vi "Read.vi"(8 "error in":errorcluster, 11 "Channel":u16) -> (0 "error out":errorcluster, 2 "MessageBuffer out":T1, 3 "Channel out":u16, 5 "function return":u32)   [LabVIEW 2025, in "PCAN API.lvlib"]
doc: "This VI is used for reading a CAN message with decoding errors from function return."
uses:
  PCAN API.lvlib
  <vilib>/Utility/file.llb/Write Delimited Spreadsheet (string).vi
  PCAN2023/PCAN2023.lvlib
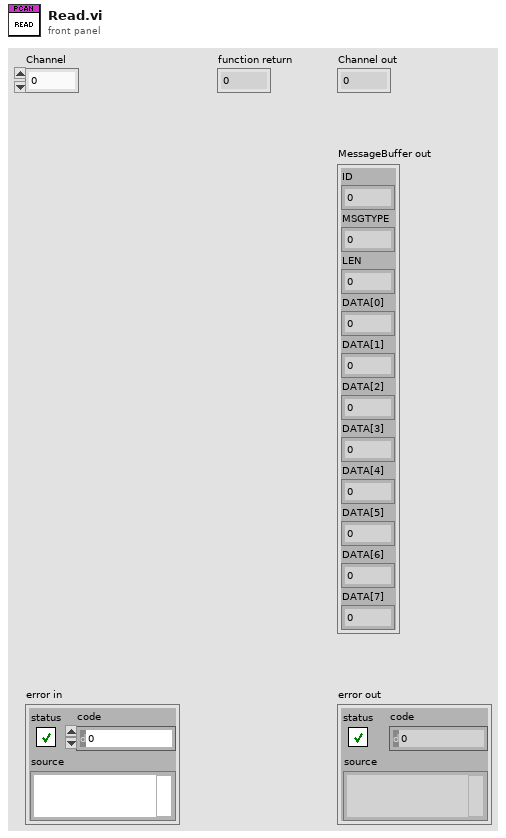
[diagram p1: front panel]
types:
  T1 = cluster{"ID":u32, "MSGTYPE":u8, "LEN":u8, "DATA[0]":u8, "DATA[1]":u8, "DATA[2]":u8, "DATA[3]":u8, "DATA[4]":u8, "DATA[5]":u8, "DATA[6]":u8, "DATA[7]":u8}
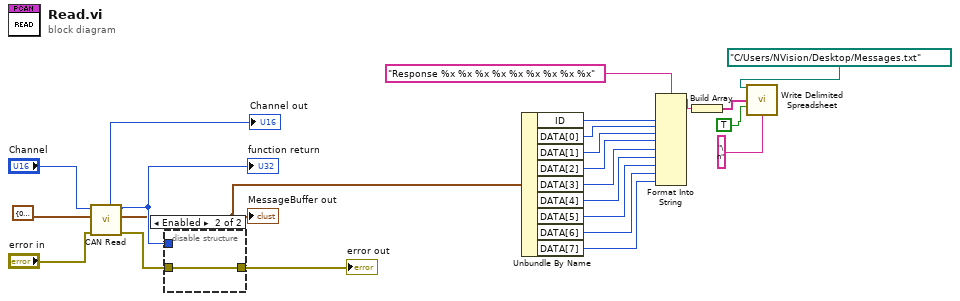
[diagram p0: block diagram]
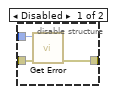
[diagram p2: hidden frame]
diagram:
  n1 = call "CAN Read.vi"("error in"="error in", "MessageBuffer"=T1 {"ID"=0, "MSGTYPE"=0, "LEN"=0, "DATA[0]"=0, "DATA[1]"=0, "DATA[2]"=0, "DATA[3]"=0, "DATA[4]"=0, "DATA[5]"=0, "DATA[6]"=0, "DATA[7]"=0}, "Channel"="Channel") -> ("error out"=w18:errorcluster, "MessageBuffer out"=w16:T1, "function return"=w19:u32, "Channel out"=→"Channel out":u16)  [unwired: 4 in, 1 out]
  "function return" <- w19
  "MessageBuffer out" <- w16
  n2 = disable-structure shown="Enabled" {
    disable-tunnel: w19 -> [w26 _]
    disable-tunnel: w18 -> [w25 w27]
    disable-tunnel: [w24 w27] -> w17
    frame Disabled {
      n3 = call "Get Error.vi"("error in (no error)"=w25, "function return"=w26) -> ("error out"=w24:errorcluster)  [unwired: 9 in]
    }
    frame Enabled {
    }
  }
  "error out" <- w17
  n4 = Unbundle By Name(w16) -> ("ID"=w14:u32, "DATA[0]"=w13:u8, "DATA[1]"=w12:u8, "DATA[2]"=w11:u8, "DATA[3]"=w10:u8, "DATA[4]"=w9:u8, "DATA[5]"=w8:u8, "DATA[6]"=w7:u8, "DATA[7]"=w6:u8)
  n5 = Format Into String(format string="Response %x %x %x %x %x %x %x %x %x", w14, w13, w12, w11, w10, w9, w8, w7, w6) -> (resulting string=w2:string)  [unwired: 2 in, 1 out]
  n6 = Build Array(w2) -> (w1:string[])
  n7 = call-poly <vilib>:"Write Delimited Spreadsheet.vi"("file path (dialog if empty)"=path "C:/Users/NVision/Desktop/Messages.txt", "1D data"=w1, "append to file? (new file:F)"=TRUE, "delimiter (\\t)"="\n" ("delimiter (\\t)")) -> ()  [unwired: 10 in, 2 out]
